vi "Disconnect.vi"(8 "error in":errorcluster, 11 "89XX in":refnum<class "89XX.lvclass">) -> (0 "error out":errorcluster, 3 "89XX out":refnum<class "89XX.lvclass">)   [LabVIEW 2019, in "89XX.lvlib" / "89XX.lvclass"]
uses:
  Library/89XX.lvclass
  Library/89XX.lvclass/89XX.ctl
  builds/Instruments/PowerSupply.lvlibp/Library/PowerSupply.lvclass
  <instrlib>/Keysight N8900 Series/Keysight N8900 Series.lvlib
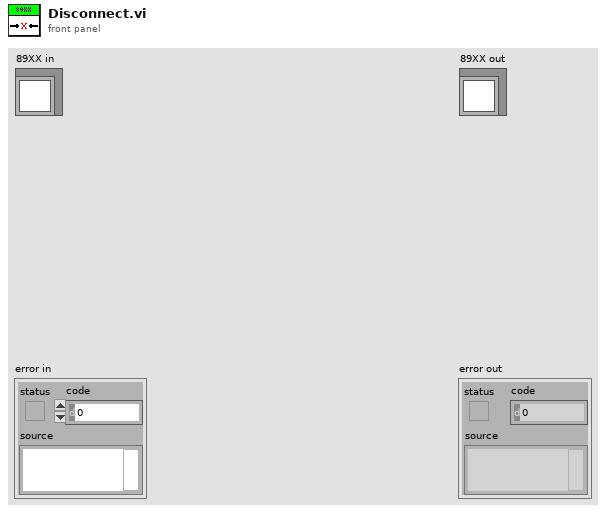
[diagram p1: front panel]
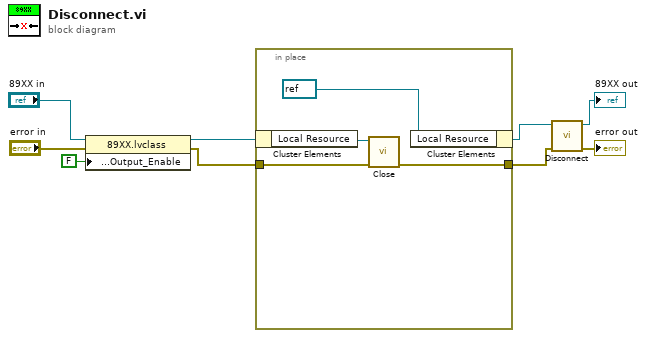
[diagram p0: block diagram]
diagram:
  n1 = property class="89XX.lvclass"(reference="89XX in", error in="error in", "Accessors:Setting:Output_Enable"=FALSE ("Supply:Settings:Output_Enable")) -> (reference out=w4:refnum<class "89XX.lvclass">, error out=w2:errorcluster)
  n2 = in-place {
    in-place-border: w2 -> [w11]
    in-place-border: [w10] -> w1
    n3 = in-place-cluster #1(w4) -> ("Local Resource"=w12:refnum<visa-resource-name>)
    n4 = call <instrlib>:"Close.vi"("error in (no error)"=w11, "VISA resource name"=w12) -> ("error out"=w10:errorcluster)  [unwired: 9 in]
    n5 = in-place-cluster #1("Local Resource"=refnum<visa-resource-name> refnum) -> (w3:refnum<class "89XX.lvclass">)
  }
  n6 = call-parent "Disconnect.vi"("error in"=w1, "Instruments in"=w3) -> ("error out"=→"error out":errorcluster, "Instruments out"=→"89XX out":refnum<class "89XX.lvclass">)  [unwired: 8 in]
